vi "Get Project Root.vi"(8 "error in (no error)":errorcluster, 11 "Project in":refnum<vi>) -> (0 "error out":errorcluster, 2 "Root":refnum<vi>, 3 "Project out":refnum<vi>)   [LabVIEW 2019, in "VI Scripting Tools.lvlib"]
uses:
  VI Scripting Tools.lvlib
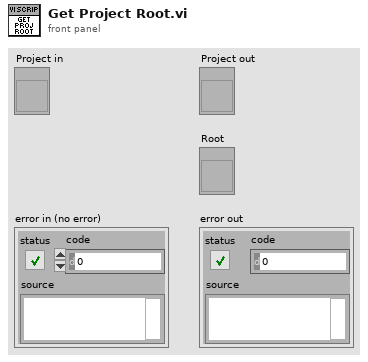
[diagram p1: front panel]
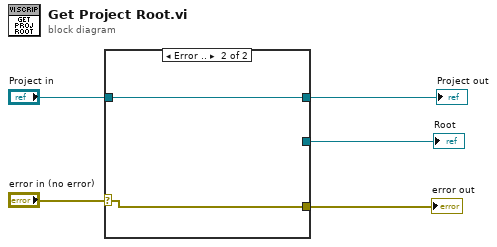
[diagram p0: block diagram]
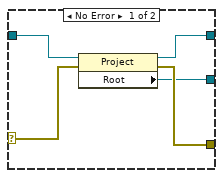
[diagram p2: hidden frame]
diagram:
  n1 = case shown="Error .." "error in (no error)" {
    selector: "error in (no error)" -> [w6 w11]
    tunnel: [w10 w11] -> w5
    tunnel: [w9 _] -> w4
    tunnel: "Project in" -> [w8 w12]
    tunnel: [w7 w12] -> w2
    frame No Error {
      n2 = property class="Project"(reference=w8, error in=w6) -> (reference out=w7:refnum<vi>, error out=w10:errorcluster, "Root"=w9:refnum<vi>)
    }
    frame Error {
    }
  }
  "error out" <- w5
  "Root" <- w4
  "Project out" <- w2
